vi "DT_Triangle Manager_Get Oppo Edge.vi"(11 "point idx":i32) -> (2 "oppo point idx 2":i32, 3 "oppo point idx 1":i32)   [LabVIEW 2017, in "NI_AAL_Geometry.lvlib"]
uses:
  <vilib>/Analysis/NI_AAL_Geometry.lvlib
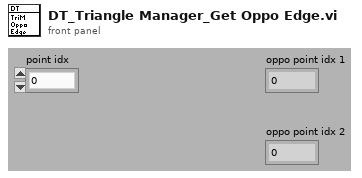
[diagram p1: front panel]
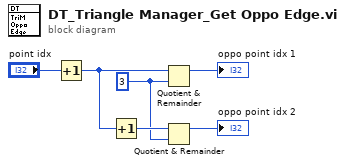
[diagram p0: block diagram]
diagram:
  w2 = 3 ("y")
  n1 = Increment(x="point idx") -> (x+1=w4:i32)
  n2 = Increment(x=w4) -> (x+1=w3:i32)
  n3 = Quotient & Remainder(x=w4, y=w2) -> (x-y*floor(x/y)=→"oppo point idx 1":i32)  [unwired: 1 out]
  n4 = Quotient & Remainder(x=w3, y=w2) -> (x-y*floor(x/y)=→"oppo point idx 2":i32)  [unwired: 1 out]
